vi "kalman pv cycle.vi"(10 "position measurement":i16, 11 "Kalman PV state":T1) -> (3 "kalman pv state out":T1)   [LabVIEW 2010]
uses:
  kalman pv state.ctl
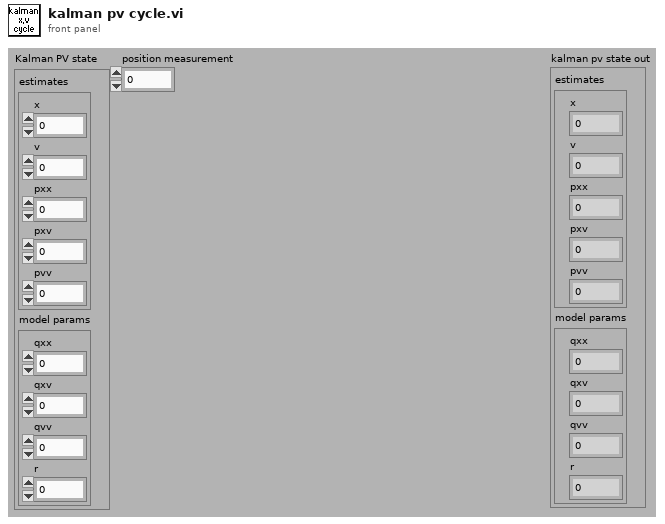
[diagram p1: front panel]
types:
  T1 = typedef "kalman pv state.ctl" = cluster{"estimates":cluster{"x":fxp<+/-,18,16>, "v":fxp<+/-,18,16>, "pxx":u16, "pxv":u16, "pvv":u16}, "model params":cluster{"qxx":u16, "qxv":u16, "qvv":u16, "r":u16}}
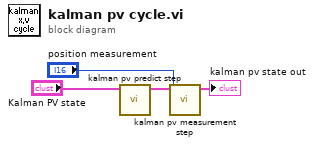
[diagram p0: block diagram]
diagram:
  n1 = call "kalman pv predict step.vi"("Kalman PV state"="Kalman PV state") -> ("Kalman PV state out"=w4:T1)  [unwired: 10 in]
  n2 = call "kalman pv measurement step.vi"("position measurement"="position measurement", "Kalman PV state"=w4) -> ("kalman pv state out"=→"kalman pv state out":T1)  [unwired: 9 in]
